vi "Excel Num to Cell.vi"(3 "Column":i32=1, 5 "Row":i32=1) -> (1 "Cell":string)   [LabVIEW 2016, in "excel.lvlib"]
uses:
  excel.lvlib
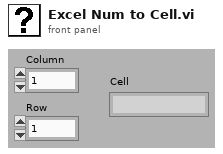
[diagram p1: front panel]
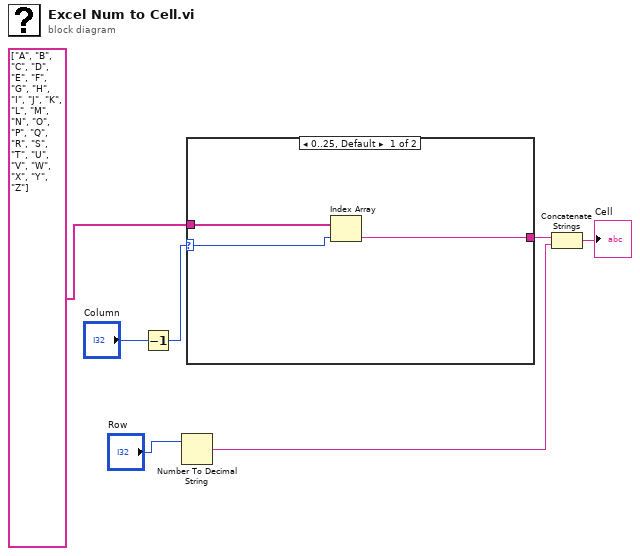
[diagram p0: block diagram]
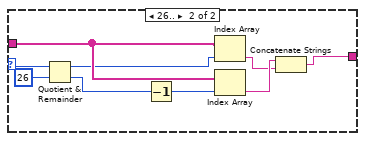
[diagram p2: hidden frame]
diagram:
  n1 = Decrement(x="Column") -> (x-1=w1:i32)
  n2 = Number To Decimal String(number="Row") -> (decimal integer string=w4:string)  [unwired: 1 in]
  n3 = case shown="0..25, Default" w1 {
    selector: w1 -> [w8 w12]
    tunnel: string[] ["A", "B", "C", "D", "E", "F", "G", "H", "I", "J", "K", "L", "M", "N", "O", "P", "Q", "R", "S", "T", "U", "V", "W", "X", "Y", "Z"] -> [w10 w17]
    tunnel: [w9 w15] -> w6
    frame 0..25, Default {
      n4 = Index Array(array=w10, index=w8) -> (element=w9:string)
    }
    frame 26.. {
      n5 = Quotient & Remainder(x=w12, y=26) -> (x-y*floor(x/y)=w16:i32, floor(x/y)=w18:i32)
      n6 = Decrement(x=w18) -> (x-1=w11:i32)
      n7 = Index Array(array=w17, index=w16) -> (element=w13:string)
      n8 = Index Array(array=w17, index=w11) -> (element=w14:string)
      n9 = Concatenate Strings(w14, w13) -> (w15:string)
    }
  }
  n10 = Concatenate Strings(w6, w4) -> (→"Cell":string)
